vi "WiiMote Graph Accelerometer.vi"() -> ()   [LabVIEW 2012]
doc: "This VI shows how to read accelerometer data from a Nintendo WiiMote."
uses:
  <vilib>/LabVIEW Hacker/WiiMote/WiiMote State.ctl
panel:
  out "Wiimote State":T1
  out "Acceleration (calibrated)":cluster{"[0]":sgl, "[1]":sgl, "[2]":sgl}(graph)
  in  "stop":bool
  # "Accelerometers"
  # "Buttons"
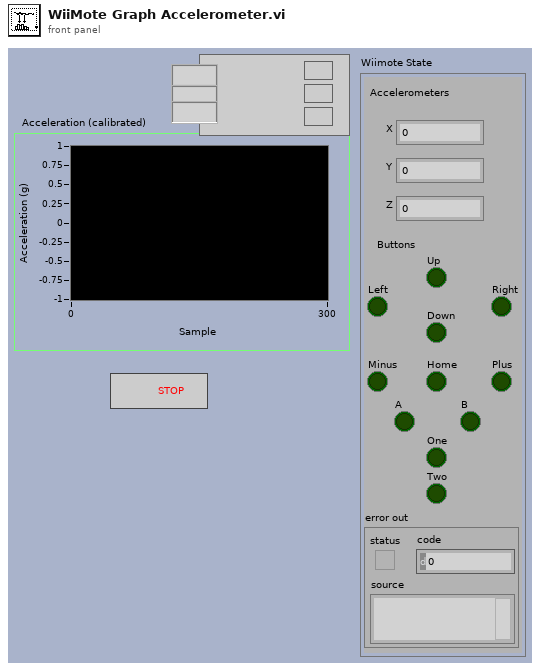
[diagram p1: front panel]
types:
  T1 = typedef "WiiMote State.ctl" = cluster{"X":sgl, "Y":sgl, "Z":sgl, "A":bool, "B":bool, "Down":bool, "Home":bool, "Left":bool, "Minus":bool, "One":bool, "Plus":bool, "Right":bool, "Two":bool, "Up":bool, "error out":errorcluster}
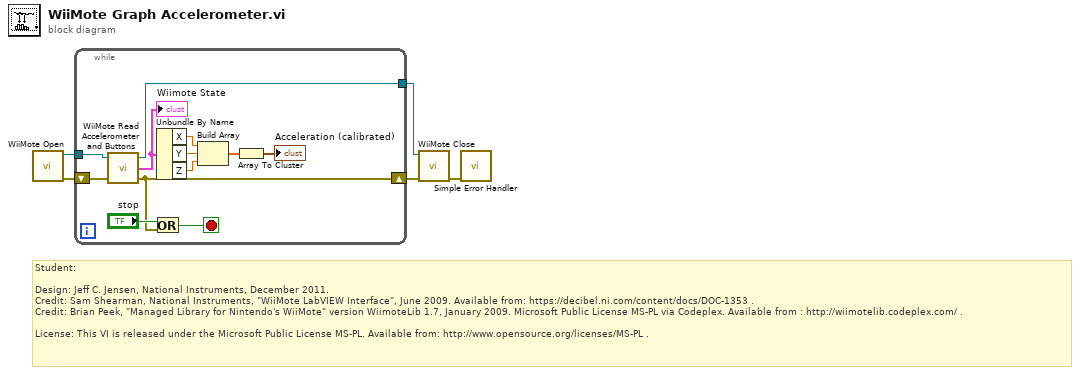
[diagram p0: block diagram]
diagram:
  # "Student: \n\nDesign: Jeff C. Jensen, National Instruments, December 2011.\nCredit: Sam Shearman, National Instruments, \"WiiMote LabVIEW Interface\", June 2009. Available from: https://decibel.ni.com/content/docs/DOC-1353 .\nCredit: Brian Peek, \"Managed Library for Nintendo's WiiMote\" version WiimoteLib 1.7, January 2009. Microsoft Public License MS-PL via Codeplex. Available from : http://wiimotelib.codeplex.com/ .\n\nLicense: This VI is released under the Microsoft Public License MS-PL. Available from: http://www.opensource.org/licenses/MS-PL ."
  n1 = call <vilib>:"WiiMote Open.vi"() -> ("error out"=w5:errorcluster, "WiiMote reference"=w2:refnum<k24>)  [unwired: 10 in]
  n2 = while {
    tunnel: w2 -> [w16]
    shift-right: [w7] -> w4
    shift-left: w5 -> [w15]
    tunnel: [w6] -> w1
    stop <- w17 stop-if-true
    n3 = call <vilib>:"WiiMote Read Accelerometer and Buttons.vi"("error in"=w15, "Wiimote"=w16) -> ("error out"=w7:errorcluster, "Wiimote State"=w14:T1, "reference out"=w6:refnum<k24>)  [unwired: 1 in]
    "Wiimote State" <- w14
    n4 = Or(x="stop", y=w7) -> (x .or. y?=w17:bool)
    n5 = Unbundle By Name(w14) -> ("X"=w12:sgl, "Y"=w10:sgl, "Z"=w11:sgl)
    n6 = Build Array(w12, w10, w11) -> (w8:sgl[])
    n7 = Array To Cluster(array=w8) -> (cluster=→"Acceleration (calibrated)":cluster{"[0]":sgl, "[1]":sgl, "[2]":sgl})
  }
  n8 = call <vilib>:"WiiMote Close.vi"("error in (no error)"=w4, "wiimote reference"=w1) -> ("error out"=w3:errorcluster)  [unwired: 9 in]
  n9 = call <vilib>:"Simple Error Handler.vi"("error in (no error)"=w3) -> ()  [unwired: 4 in, 5 out]
